vi "SUB_IMM 영문 모드로 변경.vi"(11 "프런트패널 윈도우:제목":string) -> ()   [LabVIEW 2015]
uses:
  imm32.dll
panel:
  out "Sentence":i64
  out "Conversion":i64
  # "Alphanumeric input mode. This is the default, defined as 0x0000."
  # "// C++ 코드 \nvoid __fastcall ToggleHanMode(void) \n{ \n    unsigned long Conversion, Sentence; \n    HIMC Mode = ImmGetContext(Application->Handle); \n    ImmGetConversionStatus(Mode, &Conversion, &Sentence); \n    if (Conversion == IME_CMODE_HANGEUL) \n        ImmSetConversionStatus(Mode, IME_CMODE_ALPHANUMERIC, IME_CMODE_ALPHANUMERIC); \n    else \n        ImmSetConversionStatus(Mode, IME_CMODE_HANGEUL, IME_CMODE_HANGEUL); \n} \n\n[출처] 한영 입력상태 알아내기 및 전환하기 |작성자 무한별"
  # "// C++ 코드 \nbool __fastcall GetHanMode(void) \n{ \n    unsigned long Conversion, Sentence; \n    HIMC Mode = ImmGetContext(Application->Handle); \n    ImmGetConversionStatus(Mode, &Conversion, &Sentence); \n    return (Conversion == IME_CMODE_HANGEUL); \n} \n\n[출처] 한영 입력상태 알아내기 및 전환하기 |작성자 무한별"
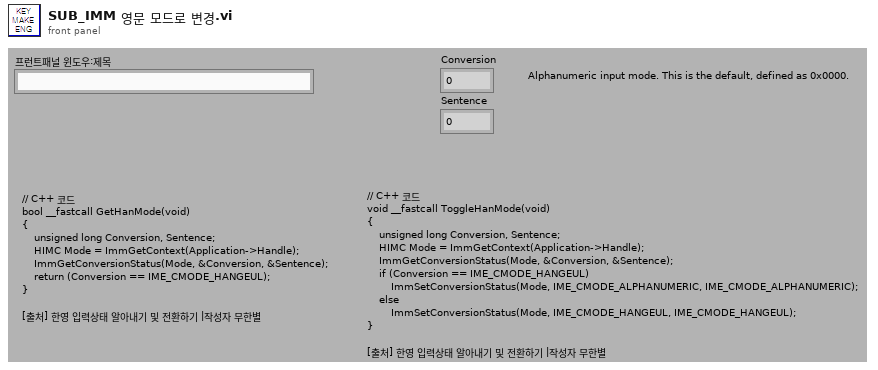
[diagram p1: front panel]
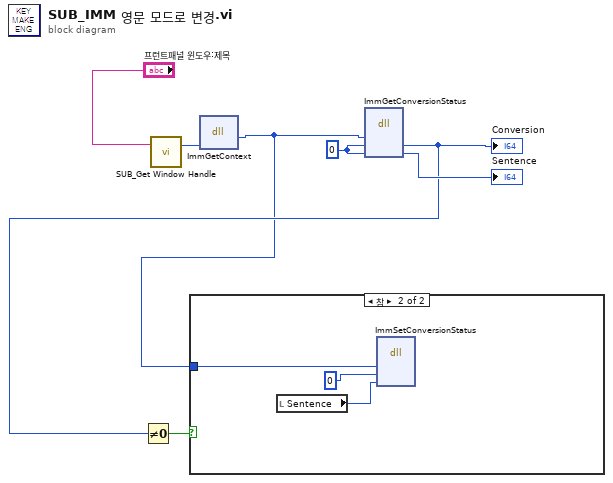
[diagram p0: block diagram]
diagram:
  w5 = i64 0 ("HKL")
  n1 = call "SUB_Get Window Handle.vi"("Window Name"="프런트패널 윈도우:제목") -> ("Window Handle"=w6:i32)  [unwired: 2 in]
  n2 = dll-call lib="imm32.dll" fn="ImmGetContext"("hWnd"=w6) -> ("return type"=w1:i32)  [unwired: 4 in, 2 out]
  n3 = dll-call lib="imm32.dll" fn="ImmGetConversionStatus"("hIMC"=w1, "Conversion"=w5, "Sentence"=w5) -> ("Conversion"=w3:u32, "Sentence"=→"Sentence":u32)  [unwired: 5 in, 2 out]
  "Conversion" <- w3
  n4 = Not Equal To 0?(x=w3) -> (x != 0?=w2:bool)
  n5 = case shown="참" w2 {
    tunnel: w1 -> [_ w10]
    frame False {
    }
    frame True {
      n6 = local read "Sentence"() -> (w8:i64)
      n7 = dll-call lib="imm32.dll" fn="ImmSetConversionStatus"("hIMC"=w10, "Conversion"=i64 0 ("HKL"), "Sentence"=w8) -> ()  [unwired: 7 in, 2 out]
    }
  }
